vi "temp.vi"() -> (0 "Thermometer":dbl(slide) scale=0.0..100.0, 1 "32bit integer":i32)   [LabVIEW 2018]
doc: "This VI simulates acquiring temperature data one value at a time. The temperature is displayed in degrees Fahrenheit."
panel:
  out "Numeric":dbl
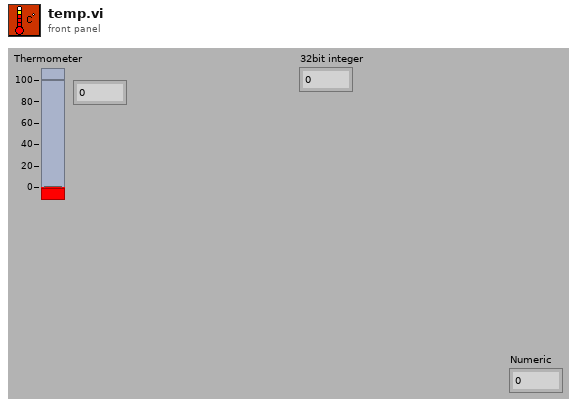
[diagram p1: front panel]
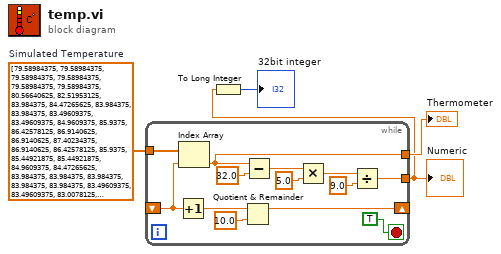
[diagram p0: block diagram]
diagram:
  w4 = dbl[] [79.58984375, 79.58984375, 79.58984375, 79.58984375, 79.58984375, 79.58984375, 80.56640625, 82.51953125, 83.984375, 84.47265625, 83.984375, 83.984375, 83.49609375, 83.49609375, 84.9609375, 85.9375, 86.42578125, 86.9140625, 86.9140625, 87.40234375, 86.9140625, 86.42578125, 85.9375, 85.44921875, 85.44921875, 84.9609375, 84.47265625, 83.984375, 83.984375, 83.984375, 83.984375, 83.984375, 83.49609375, 83.49609375, 83.0078125, 83.0078125, 83.0078125, 83.984375, 84.47265625, 84.9609375, 85.44921875, 86.42578125, 86.9140625, 86.9140625, 86.9140625, 86.42578125, 85.9375, 85.44921875, 85.9375, 86.9140625, 87.40234375, 87.890625, 87.40234375, 86.9140625, 86.9140625, 85.9375, 85.9375, 85.9375, 84.9609375, 84.9609375, 84.9609375, 84.47265625, 84.47265625, 85.44921875, 85.9375, 86.9140625, 86.9140625, 86.42578125, 85.9375, 85.44921875, 85.44921875, 84.9609375, 84.9609375, 84.47265625, 84.47265625, 83.984375, 83.984375, 83.49609375, 83.49609375, 83.0078125, 83.0078125, 83.0078125, 83.0078125, 83.0078125, 83.0078125, 83.0078125, 82.51953125, 81.0546875, 81.54296875, 82.51953125, 83.0078125, 82.51953125, 82.03125, 82.03125, 82.03125, 82.03125, 81.54296875, 81.54296875, 81.54296875, 81.54296875]  # Simulated Temperature
  n1 = while {
    tunnel: w4 -> [w13]
    tunnel: [w6] -> w3
    shift-left: _ -> [w17]
    shift-right: [w14] -> _
    tunnel: [w5] -> w2
    stop <- TRUE stop-if-true
    n2 = Increment(x=w17) -> (x+1=w16:dbl)
    n3 = Index Array(array=w13, index=w17) -> (element=w6:dbl)
    n4 = Quotient & Remainder(x=w16, y=10.0) -> (x-y*floor(x/y)=w14:dbl)  [unwired: 1 out]
    n5 = Subtract(x=w6, y=32.0) -> (x-y=w10:dbl)
    n6 = Multiply(x=w10, y=5.0) -> (x*y=w9:dbl)
    n7 = Divide(x=w9, y=9.0) -> (x/y=w5:dbl)
  }
  "Thermometer" <- w3
  "Numeric" <- w2
  n8 = To Long Integer(number=w2) -> (32bit integer=→"32bit integer":i32)
